vi "Automatic Assembly DB.vi"() -> ()   [LabVIEW 2021]
uses:
  Classes/Assembly/Database Entry/Database Entry.lvclass
  Classes/Assembly/Assembly Run.lvclass
  <vilib>/Utility/file.llb/Read Delimited Spreadsheet (string).vi
  SubVIs/PUT_region.vi
  SubVIs/component_tray_region.vi
  SubVIs/assembly_tray_region.vi
  Classes/Controller/I-O/I-O.lvclass
  Classes/Controller/Controller.lvclass
panel:
  in  "Abort assembly":bool
  in  "Do old-style single-module data-entry?":bool
  out "Status":string
  out "Stack names":T1
  out "Feet check":bool
  out "Assembly Type":string
  out "Assembly tray region":dbl
  out "Component tray region":dbl
  out "PUT Region":dbl
  # "Click the Run arrow to start.\nFill out pop-up prompts.\nSee Status for more info.\nAnswer ALL prompts until program stops running!"
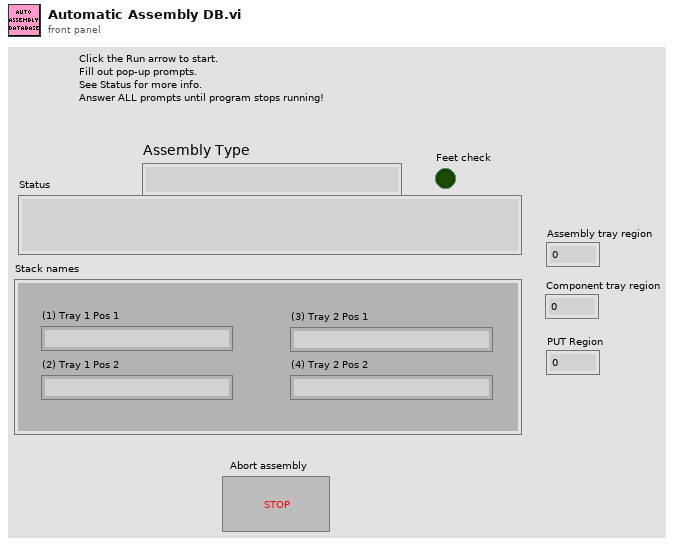
[diagram p1: front panel]
types:
  T1 = cluster{"(1) Tray 1 Pos 1":string, "(2) Tray 1 Pos 2":string, "(3) Tray 2 Pos 1":string, "(4) Tray 2 Pos 2":string}
  T2 = enum8{"Enabled", "Disabled", "Disabled and Grayed Out"}
  T3 = typedef "File Paths.ctl" = cluster{"Glue Pattern Folder":path, "Carrier Tray Folder":path, "Pick Up Tool Fixture Folder":path, "Components Folder":path, "Bellows Tool Offset.txt":path, "Pick Up Tool Offset.txt":path, "Dispense Tip Offset.txt":path, "Log Files":path, "Gantry Assembly Map.txt":path, "Syringe and offset map.txt":path, "Controllers Folder":path, "Local dbase config":path}
  T4 = typedef "Controller.lvclass/Controllers.ctl" = cluster{"I-O.lvclass":refnum<class "I-O.lvclass">, "Gantry":refnum<k24>, "Dispenser":refnum<visa-resource-name>}
  T5 = cluster{"Fixture ID":dbl, "Position":dbl, "Thickness":dbl}[]
  T6 = cluster{"Stack names[0]":string, "Stack names[1]":string, "Stack names[2]":string, "Stack names[3]":string}
  T7 = cluster{"Fixture ID":dbl, "Position":dbl, "Thickness":dbl}[][]
  T8 = cluster{"Fixture ID":dbl, "Position":dbl, "Thickness":dbl}
  T9 = typedef "I-O.lvclass/Pin Map.ctl" = cluster{"Region Valves":i32[], "Extra Valves":dbl[][][], "Tool Primary Valve":i32, "Tool Secondary Valve":i32, "Region Sensors":i32[], "Extra Sensors":dbl[][][], "Tool Primary Sensor":dbl, "Tool Secondary Sensor":dbl, "Compression Sensor":dbl, "5V":i32, "Dispenser Sensor":dbl}
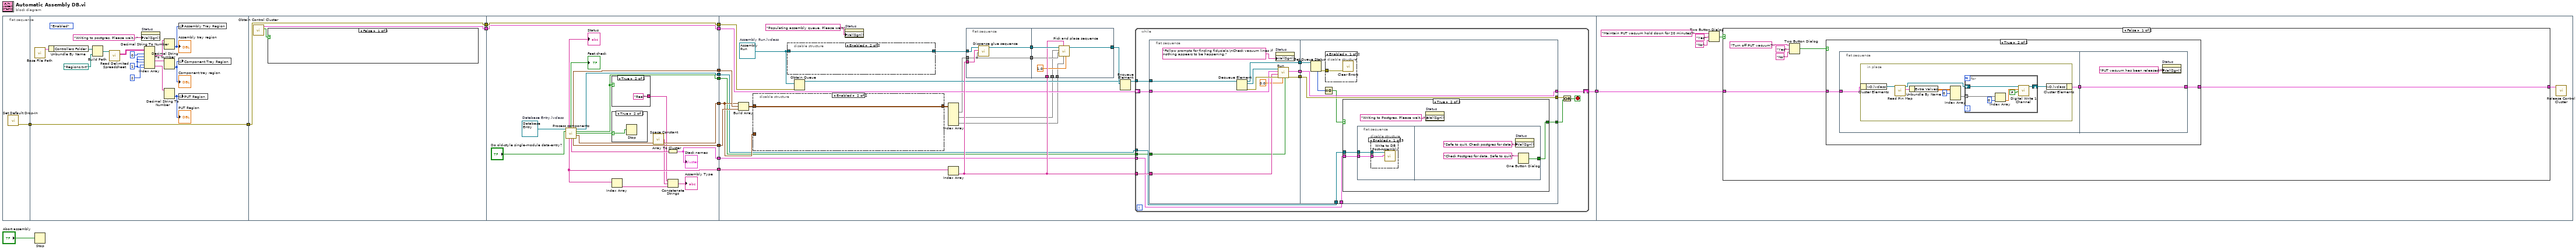
[diagram p0: block diagram]
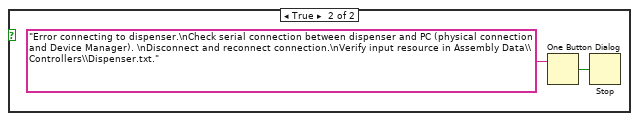
[diagram p2: hidden frame]
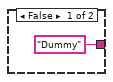
[diagram p3: hidden frame]
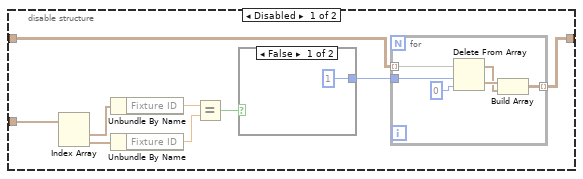
[diagram p5: hidden frame]
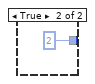
[diagram p6: hidden frame]
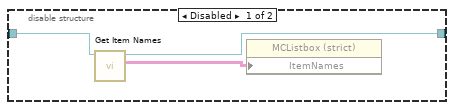
[diagram p7: hidden frame]
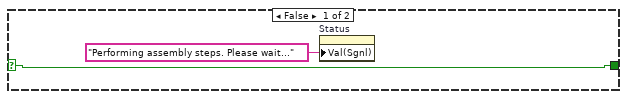
[diagram p9: hidden frame]
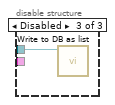
[diagram p11: hidden frame]
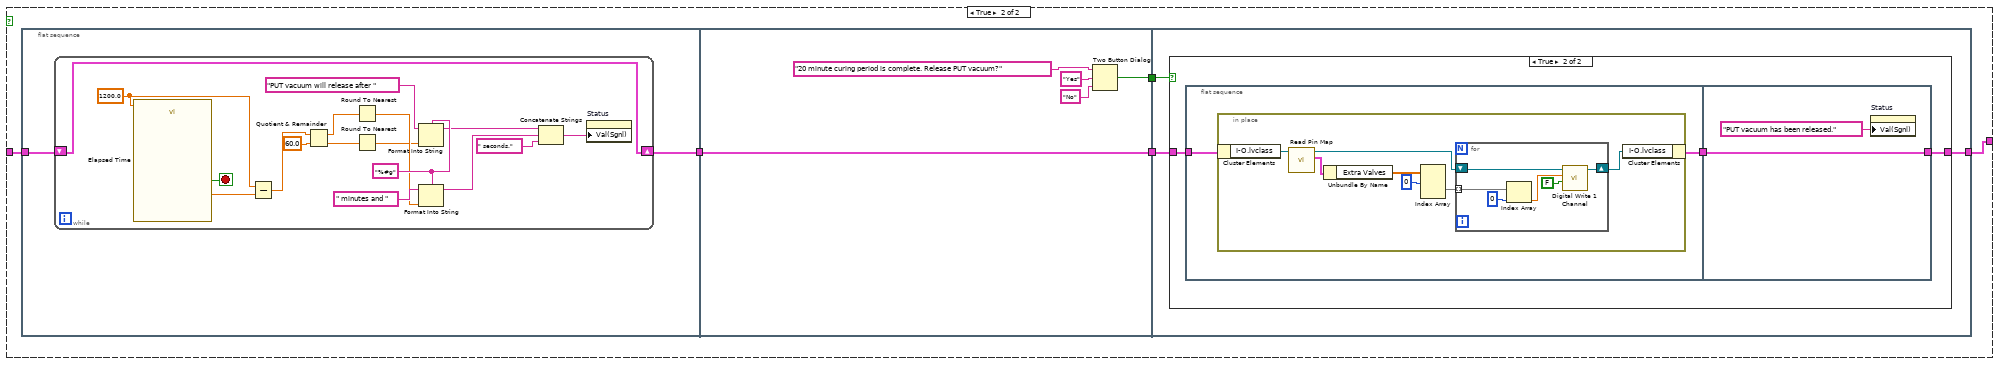
[diagram p13: hidden frame]
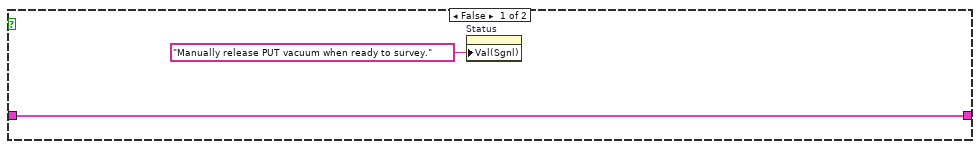
[diagram p14: hidden frame]
diagram:
  n1 = flat-sequence {
    tunnel: [w16] -> w14
    tunnel: [w18] -> w7
    tunnel: w14 -> [w18]
    tunnel: w7 -> [w35]
    tunnel: [w35] -> w6
    tunnel: [w33] -> w4
    tunnel: [w55] -> w15
    tunnel: w6 -> [w55]
    tunnel: [w54] -> w13
    tunnel: [w53] -> w12
    tunnel: [w52] -> w11
    tunnel: [w44] -> w10
    tunnel: [w48] -> w9
    tunnel: [w46] -> w8
    tunnel: [w39] -> w5
    tunnel: w4 -> [w39]
    tunnel: [w38] -> w1
    tunnel: w15 -> [w82]
    tunnel: w13 -> [w81]
    tunnel: w12 -> [w80]
    tunnel: w11 -> [w76]
    tunnel: w10 -> [w79]
    tunnel: w9 -> [w73]
    tunnel: w8 -> [w74]
    tunnel: w5 -> [w75]
    tunnel: [w64] -> w2
    tunnel: w1 -> [w60]
    tunnel: w2 -> [w170]
    frame #0 {
      n2 = call "Set Default Drop-In.vi"() -> ("error out"=w16:errorcluster)  [unwired: 11 in]
    }
    frame #1 {
      (unwired) T2."Enabled" ("Disabled")
      w21 = 1 ("disabled index (col)")
      n3 = call "Base File Path.vi"() -> ("Paths Out"=w32:T3)  [unwired: 11 in]
      n4 = Unbundle By Name(w32) -> ("Controllers Folder"=w30:path)
      n5 = Build Path(base path=w30, name or relative path=path "Regions.txt") -> (appended path=w31:path)
      n6 = call-poly <vilib>:"Read Delimited Spreadsheet.vi"("file path (dialog if empty)"=w31) -> ("all rows"=w19:string[][])  [unwired: 9 in, 5 out]
      n7 = property on="Status" class="Str"("Val(Sgnl)"="Writing to postgres. Please wait..." ("Value (Signaling)")) -> ()  [unwired: 2 in, 2 out]
      n8 = Index Array(array=w19, index (row) #1=0 ("index (row)"), index (col) #1=w21, index (row) #2=w21, index (col) #2=w21, index (row) #3=2 ("disabled index (row)"), index (col) #3=w21) -> (element #1=w24:string, element #2=w23:string, element #3=w25:string)
      n9 = Decimal String To Number(string=w24) -> (number=w27:i32)  [unwired: 2 in, 1 out]
      "Assembly tray region" <- w27
      n10 = Decimal String To Number(string=w23) -> (number=w28:i32)  [unwired: 2 in, 1 out]
      "Component tray region" <- w28
      n11 = Decimal String To Number(string=w25) -> (number=w26:i32)  [unwired: 2 in, 1 out]
      "PUT Region" <- w26
      n12 = global write "assembly_tray_region.vi" "Assembly Tray Region"(w27) -> ()
      n13 = global write "component_tray_region.vi" "Component Tray Region"(w28) -> ()
      n14 = global write "PUT_region.vi" "PUT Region"(w26) -> ()
    }
    frame #2 {
      n15 = call "Obtain Control Cluster.vi"() -> ("Dispenser error?"=w34:bool, "Control Out"=w33:T4)  [unwired: 10 in]
      n16 = case shown="False" w34 {
        frame False {
        }
        frame True {
          n17 = One Button Dialog(message="Error connecting to dispenser.\nCheck serial connection between dispenser and PC (physical connection and Device Manager). \nDisconnect and reconnect connection.\nVerify input resource in Assembly Data\\Controllers\\Dispenser.txt.") -> (true=w36:bool)  [unwired: 1 in]
          n18 = Stop(stop? (T)=w36) -> ()
        }
      }
    }
    frame #3 {
      w56 = refnum<class "Database Entry.lvclass"> refnum  # Database Entry.lvclass
      n19 = call "Process components.vi"("Database Entry in"=w56, "Do single-module data entry?"="Do old-style single-module data-entry?") -> ("Status"=→"Status":string, "Feet check"=→"Feet check":bool, "PUT Settings"=w53:T5, "Database Entry out"=w46:refnum<class "Database Entry.lvclass">, "Is real run?"=w38:bool, "Aborted"=w49:bool, "Assembly Settings"=w52:T5, "Assembly Type"=w44:string[], "Stack names"=w51:string[], "Component Settings"=w54:T5)  [unwired: 3 in, 1 out]
      n20 = case shown="True" w38 {
        tunnel: ["Dummy" "Real"] -> w41
        frame False {
        }
        frame True {
        }
      }
      n21 = case shown="True" w49 {
        selector: w49 -> [_ w59]
        frame False {
        }
        frame True {
          n22 = Stop(stop? (T)=w59) -> ()
        }
      }
      n23 = Index Array(array=w44) -> (element=w43:string)  [unwired: 1 in]
      n24 = call <vilib>:"Space Constant.vi"() -> ("String"=w42:string)
      n25 = Array To Cluster(array=w51) -> (cluster=w48:T6)
      "Stack names" <- w48
      n26 = Concatenate Strings(w41, w42, w43) -> (→"Assembly Type":string)
    }
    frame #4 {
      w83 = refnum<class "Assembly Run.lvclass"> refnum  # Assembly Run.lvclass
      n27 = Build Array(w76, w80, w81) -> (w70:T7)
      n28 = disable-structure shown="Enabled" {
        disable-tunnel: w76 -> [w103 _]
        disable-tunnel: [w102 w112] -> w71
        disable-tunnel: w70 -> [w101 w112]
        frame Disabled {
          n29 = Index Array(array=w103) -> (element #1=w100:T8, element #2=w99:T8)  [unwired: 2 in]
          n30 = Unbundle By Name(w100) -> ("Fixture ID"=w98:dbl)
          n31 = Unbundle By Name(w99) -> ("Fixture ID"=w97:dbl)
          n32 = Equal?(x=w98, y=w97) -> (x = y?=w96:bool)
          n33 = case shown="False" w96 {
            tunnel: [1 2] -> w95
            frame False {
            }
            frame True {
            }
          }
          n34 = for {
            tunnel: w101 -> [w111] mode=indexing
            tunnel: [w110] -> w102 mode=indexing
            tunnel: w95 -> [w106]
            n35 = Delete From Array(array=w111, length=w106, index=0) -> (deleted portion=w108:T5, array with subset deleted=w107:T5)
            n36 = Build Array(w108, w107) -> (w110:T7)
          }
        }
        frame Enabled {
        }
      }
      n37 = disable-structure shown="Enabled" {
        disable-tunnel: w83 -> [w115 w116]
        disable-tunnel: [w113 w116] -> w72
        frame Disabled {
          n38 = call "Get Item Names.vi"("Assembly Run in"=w115) -> ("Item names"=w114:string[][], "Assembly Run out"=w113:refnum<class "Assembly Run.lvclass">)  [unwired: 8 in, 1 out]
          n39 = property class="MCListbox (strict)"("ItemNames"=w114) -> ()  [unwired: 2 in, 2 out]
        }
        frame Enabled {
        }
      }
      n40 = Obtain Queue(element data type=w83, error in (no error)=w82) -> (queue out=w77:refnum<queue>)  [unwired: 3 in, 2 out]
      n41 = property on="Status" class="Str"("Val(Sgnl)"="Populating assembly queue. Please wait." ("Value (Signaling)")) -> ()  [unwired: 2 in, 2 out]
      n42 = Index Array(array=w71) -> (element #1=w69:T5, element #2=w68:T5, element #3=w67:T5)  [unwired: 6 in]
      n43 = Index Array(array=w79) -> (element=w78:string)  [unwired: 1 in]
      n44 = flat-sequence {
        tunnel: [w86] -> w63
        tunnel: w72 -> [w87]
        tunnel: w78 -> [w85]
        tunnel: w69 -> [w84]
        tunnel: [w84] -> w62
        tunnel: [w93] -> w66
        tunnel: w63 -> [w94]
        tunnel: w78 -> [w92]
        tunnel: w62 -> [w90]
        tunnel: w68 -> [w89]
        tunnel: w67 -> [w88]
        frame #0 {
          n45 = call "Dispense glue sequence.vi"("Assembly Tray Settings Array"=w84, "Assembly Type"=w85, "Assembly Run in"=w87) -> ("Assembly Run out"=w86:refnum<class "Assembly Run.lvclass">)  [unwired: 7 in, 1 out]
        }
        frame #1 {
          n46 = call "Pick and place sequence.vi"("Numeric"=1.0, "Component Tray map"=w88, "Assembly Type"=w92, "Assembly Tray map"=w90, "PUT map"=w89, "Assembly Run in"=w94) -> ("Assembly Run out"=w93:refnum<class "Assembly Run.lvclass">)  [unwired: 4 in, 1 out]
        }
      }
      n47 = Enqueue Element(queue=w77, element=w66) -> (queue out=w65:refnum<queue>)  [unwired: 2 in, 2 out]
      n48 = while {
        shift-right: [w128] -> w64
        shift-left: w75 -> [w129]
        tunnel: w78 -> [w127]
        tunnel: w65 -> [w126]
        tunnel: w74 -> [w120]
        tunnel: w73 -> [w119]
        tunnel: w60 -> [w117]
        stop <- w121 stop-if-true
        n49 = flat-sequence {
          tunnel: w129 -> [w138]
          tunnel: w127 -> [w136]
          tunnel: w126 -> [w133]
          tunnel: [w137] -> w125
          tunnel: [w135] -> w124
          tunnel: [w134] -> w123
          tunnel: w117 -> [w130]
          tunnel: [w148] -> w122
          tunnel: [w149] -> w128
          tunnel: w125 -> [w149]
          tunnel: w124 -> [w148]
          tunnel: w123 -> [w147]
          tunnel: w120 -> [w143]
          tunnel: w119 -> [w142]
          tunnel: [w141] -> w118
          frame #0 {
            n50 = Dequeue Element(queue=w133) -> (queue out=w134:refnum<queue>, element=w140:refnum<class "Assembly Run.lvclass">, error out=w139:errorcluster)  [unwired: 2 in, 1 out]
            n51 = property on="Status" class="Str"("Val(Sgnl)"="Follow prompts for finding fiducials.\nCheck vacuum lines if nothing appears to be happening." ("Value (Signaling)")) -> ()  [unwired: 2 in, 2 out]
            n52 = call-dynamic "Run.vi"("Dispense?"=w130, "Pickup_Test_Number"=0.0, "error in (no error)"=w139, "Assembly Type"=w136, "Control In"=w138, "Assembly In"=w140) -> ("error out"=w135:errorcluster, "Control Out"=w137:T4)  [unwired: 3 in, 1 out]
          }
          frame #1 {
            n53 = Get Queue Status(queue=w147) -> (error out=w144:errorcluster, # elements in queue=w146:i32)  [unwired: 2 in, 6 out]
            n54 = Equal To 0?(x=w146) -> (x = 0?=w145:bool)
            n55 = disable-structure shown="Enabled" {
              disable-tunnel: w144 -> [w150 _]
              frame Enabled {
                n56 = call <vilib>:"Clear Errors.vi"("error in (no error)"=w150) -> ()  [unwired: 5 in, 2 out]
              }
              frame Disabled {
              }
            }
            n57 = case shown="True" w145 {
              selector: w145 -> [w151 _]
              tunnel: w143 -> [_ w155]
              tunnel: w142 -> [_ w154]
              tunnel: [w151 w153] -> w141
              frame False {
                n58 = property on="Status" class="Str"("Val(Sgnl)"="Performing assembly steps. Please wait...") -> ()  [unwired: 2 in, 2 out]
              }
              frame True {
                n59 = flat-sequence {
                  tunnel: w155 -> [w158]
                  tunnel: w154 -> [w157]
                  tunnel: [w162] -> w153
                  frame #0 {
                    n60 = disable-structure shown="Enabled" {
                      disable-tunnel: w158 -> [w160 _ w161]
                      disable-tunnel: w157 -> [w159 _ _]
                      frame Enabled {
                        n61 = call "Write to DB Post-Assembly.vi"("Stack names"=w159, "Database Entry in"=w160) -> ()  [unwired: 8 in, 2 out]
                      }
                      frame Disabled {
                      }
                      frame Disabled {
                        n62 = call "Write to DB as list.vi"("Database Entry in"=w161) -> ()  [unwired: 8 in, 3 out]
                      }
                    }
                  }
                  frame #1 {
                    n63 = property on="Status" class="Str"("Val(Sgnl)"="Safe to quit. Check postgres for data.") -> ()  [unwired: 2 in, 2 out]
                    n64 = One Button Dialog(message="Check Postgres for data. Safe to quit.") -> (true=w162:bool)  [unwired: 1 in]
                  }
                }
                n65 = property on="Status" class="Str"("Val(Sgnl)"="Writing to Postgres. Please wait...") -> ()  [unwired: 2 in, 2 out]
              }
            }
          }
        }
        n66 = Or(x=w122, y=w118) -> (x .or. y?=w121:bool)
      }
    }
    frame #5 {
      n67 = Two Button Dialog(message="Maintain PUT vacuum hold down for 20 minutes?", 1:"No" ("F button name (\"Cancel\")"), 2:"Yes" ("T button name (\"OK\")")) -> (T button?=w165:bool)
      n68 = case shown="False" w165 {
        tunnel: w170 -> [w172 w202]
        tunnel: [w171 w198] -> w169
        frame False {
          n69 = Two Button Dialog(message="Turn off PUT vacuum?", 1:"No" ("F button name (\"Cancel\")"), 2:"Yes" ("T button name (\"OK\")")) -> (T button?=w173:bool)
          n70 = case shown="True" w173 {
            tunnel: w172 -> [w177 w179]
            tunnel: [w177 w178] -> w171
            frame False {
            }
            frame True {
              n71 = flat-sequence {
                tunnel: w179 -> [w182]
                tunnel: [w181] -> w180
                tunnel: w180 -> [w197]
                tunnel: [w197] -> w178
                frame #0 {
                  n72 = in-place {
                    n73 = in-place-cluster #1(w182) -> ("I-O.lvclass"=w184:refnum<class "I-O.lvclass">)
                    n74 = call-dynamic "Read Pin Map.vi"("I-O in"=w184) -> ("Pin Map 2"=w189:T9, "I-O out"=w186:refnum<class "I-O.lvclass">)  [unwired: 8 in, 1 out]
                    n75 = Unbundle By Name(w189) -> ("Extra Valves"=w188:dbl[][][])
                    n76 = Index Array(array=w188, index (dim 0)=0 ("index (page)")) -> (element=w187:dbl[][])  [unwired: 2 in]
                    n77 = for {
                      tunnel: w187 -> [w195] mode=indexing
                      shift-right: [w193] -> w183
                      shift-left: w186 -> [w194]
                      n78 = Index Array(array=w195, index=0) -> (element=w192:dbl)
                      n79 = call-dynamic "Digital Write 1 Channel.vi"("Value"=FALSE, "Channel"=w192, "I-O.lvclass"=w194) -> ("I-O.lvclass 2"=w193:refnum<class "I-O.lvclass">)  [unwired: 7 in, 1 out]
                    }
                    n80 = in-place-cluster #1("I-O.lvclass"=w183) -> (w181:T4)
                  }
                }
                frame #1 {
                  n81 = property on="Status" class="Str"("Val(Sgnl)"="PUT vacuum has been released." ("Value (Signaling)")) -> ()  [unwired: 2 in, 2 out]
                }
              }
            }
          }
        }
        frame True {
          n82 = flat-sequence {
            tunnel: w202 -> [w203]
            tunnel: [w204] -> w201
            tunnel: w201 -> [w226]
            tunnel: [w226] -> w200
            tunnel: [w223] -> w199
            tunnel: w200 -> [w228]
            tunnel: w199 -> [w229]
            tunnel: [w227] -> w198
            frame #0 {
              n83 = while {
                shift-right: [w217] -> w204
                shift-left: w203 -> [w217]
                stop <- w221 stop-if-true
                w211 = "%#g" ("format string")
                w220 = 1200.0 ("Time Target (s)")
                n84 = call "Elapsed Time"("Time Target (s)"=w220) -> ("Elapsed Time (s)"=w219:dbl, "Time has Elapsed"=w221:bool)  [unwired: 11 in, 6 out]
                n85 = Subtract(x=w220, y=w219) -> (x-y=w216:dbl)
                n86 = Quotient & Remainder(x=w216, y=60.0) -> (x-y*floor(x/y)=w214:dbl, floor(x/y)=w213:dbl)
                n87 = Round To Nearest(number=w214) -> (nearest integer value=w206:dbl)
                n88 = Round To Nearest(number=w213) -> (nearest integer value=w205:dbl)
                n89 = Format Into String(format string=w211, initial string="PUT vacuum will release after ", w205) -> (resulting string=w208:string)  [unwired: 1 in, 1 out]
                n90 = Format Into String(format string=w211, initial string=" minutes and ", w206) -> (resulting string=w212:string)  [unwired: 1 in, 1 out]
                n91 = Concatenate Strings(w208, w212, " seconds." ("string")) -> (w215:string)
                n92 = property on="Status" class="Str"("Val(Sgnl)"=w215) -> ()  [unwired: 2 in, 2 out]
              }
            }
            frame #1 {
              n93 = Two Button Dialog(message="20 minute curing period is complete. Release PUT vacuum?", 1:"No" ("F button name (\"Cancel\")"), 2:"Yes" ("T button name (\"OK\")")) -> (T button?=w223:bool)
            }
            frame #2 {
              n94 = case shown="True" w229 {
                tunnel: w228 -> [w231 w234]
                tunnel: [w231 w232] -> w227
                frame False {
                  n95 = property on="Status" class="Str"("Val(Sgnl)"="Manually release PUT vacuum when ready to survey." ("Value (Signaling)")) -> ()  [unwired: 2 in, 2 out]
                }
                frame True {
                  n96 = flat-sequence {
                    tunnel: w234 -> [w236]
                    tunnel: [w235] -> w233
                    tunnel: w233 -> [w251]
                    tunnel: [w251] -> w232
                    frame #0 {
                      n97 = in-place {
                        n98 = in-place-cluster #2(w236) -> ("I-O.lvclass"=w238:refnum<class "I-O.lvclass">)
                        n99 = call-dynamic "Read Pin Map.vi"("I-O in"=w238) -> ("Pin Map 2"=w243:T9, "I-O out"=w240:refnum<class "I-O.lvclass">)  [unwired: 8 in, 1 out]
                        n100 = Unbundle By Name(w243) -> ("Extra Valves"=w242:dbl[][][])
                        n101 = Index Array(array=w242, index (dim 0)=0 ("index (page)")) -> (element=w241:dbl[][])  [unwired: 2 in]
                        n102 = for {
                          tunnel: w241 -> [w249] mode=indexing
                          shift-right: [w247] -> w237
                          shift-left: w240 -> [w248]
                          n103 = Index Array(array=w249, index=0) -> (element=w246:dbl)
                          n104 = call-dynamic "Digital Write 1 Channel.vi"("Value"=FALSE, "Channel"=w246, "I-O.lvclass"=w248) -> ("I-O.lvclass 2"=w247:refnum<class "I-O.lvclass">)  [unwired: 7 in, 1 out]
                        }
                        n105 = in-place-cluster #2("I-O.lvclass"=w237) -> (w235:T4)
                      }
                    }
                    frame #1 {
                      n106 = property on="Status" class="Str"("Val(Sgnl)"="PUT vacuum has been released." ("Value (Signaling)")) -> ()  [unwired: 2 in, 2 out]
                    }
                  }
                }
              }
            }
          }
        }
      }
      n107 = call "Release Control Cluster.vi"("output cluster"=w169) -> ()  [unwired: 11 in]
    }
  }
  n108 = Stop(stop? (T)="Abort assembly") -> ()
